vi "Format Instrument String Command.vi"(8 "error in (no error)":errorcluster, 9 "MetaData Lookup in":variant, 10 "MetaData":dbl[](array[numeric]), 11 "Command Parameters":T1) -> (0 "error out":errorcluster, 1 "MetaData Lookup out":variant, 3 "Command":string)   [LabVIEW 2019, in "Instrument Addon Engine.lvlib"]
uses:
  Instrument Addon Engine.lvlib
  Shared/Types/Command Parameters.ctl
  Shared/Types/Linked Channel Cluster.ctl
  Shared/Types/Meta Data RT Configuration Cluster.ctl
  Shared/Types/MetaData Parameters.ctl
  Shared/Types/Protocol Data Type.ctl
  Shared/Types/Metadata Channel Type.ctl
  Shared/Types/Type Cast Type.ctl
  Shared/Types/Endian.ctl
  Shared/Instrument Addon Shared.lvlib
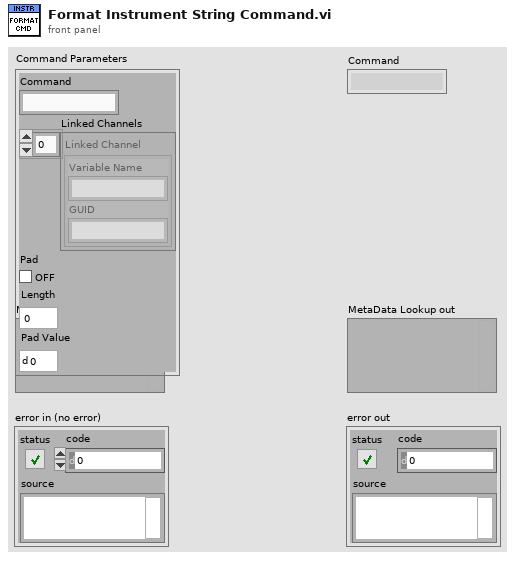
[diagram p1: front panel]
types:
  T1 = typedef "Instrument Addon Shared.lvlib/Command Parameters.ctl" = cluster{"Command":string, "Linked Channels":T2[], "Pad":bool, "Length":u32, "Pad Value":u8}
  T2 = typedef "Instrument Addon Shared.lvlib/Linked Channel Cluster.ctl" = cluster{"Variable Name":string, "GUID":string}
  T3 = typedef "Instrument Addon Shared.lvlib/Meta Data RT Configuration Cluster.ctl" = cluster{"MetaData Parameters":T4, "Data Index":i32, "Data Length":i32}
  T4 = typedef "Instrument Addon Shared.lvlib/MetaData Parameters.ctl" = cluster{"Data Type":T5, "Channel Type":T6, "List":string[], "Format String":string, "Type":T7, "Delimiter":string, "Endian":T8}
  T5 = typedef "Instrument Addon Shared.lvlib/Protocol Data Type.ctl" = enum16{"Single Channel", "Array"}
  T6 = typedef "Instrument Addon Shared.lvlib/Metadata Channel Type.ctl" = enum16{"Enumerated List", "Format", "Type Cast"}
  T7 = typedef "Instrument Addon Shared.lvlib/Type Cast Type.ctl" = enum16{"DBL", "SGL", "U64", "U32", "U16", "U8", "I64", "I32", "I16", "I8"}
  T8 = typedef "Instrument Addon Shared.lvlib/Endian.ctl" = enum16{"Native", "Little", "Big"}
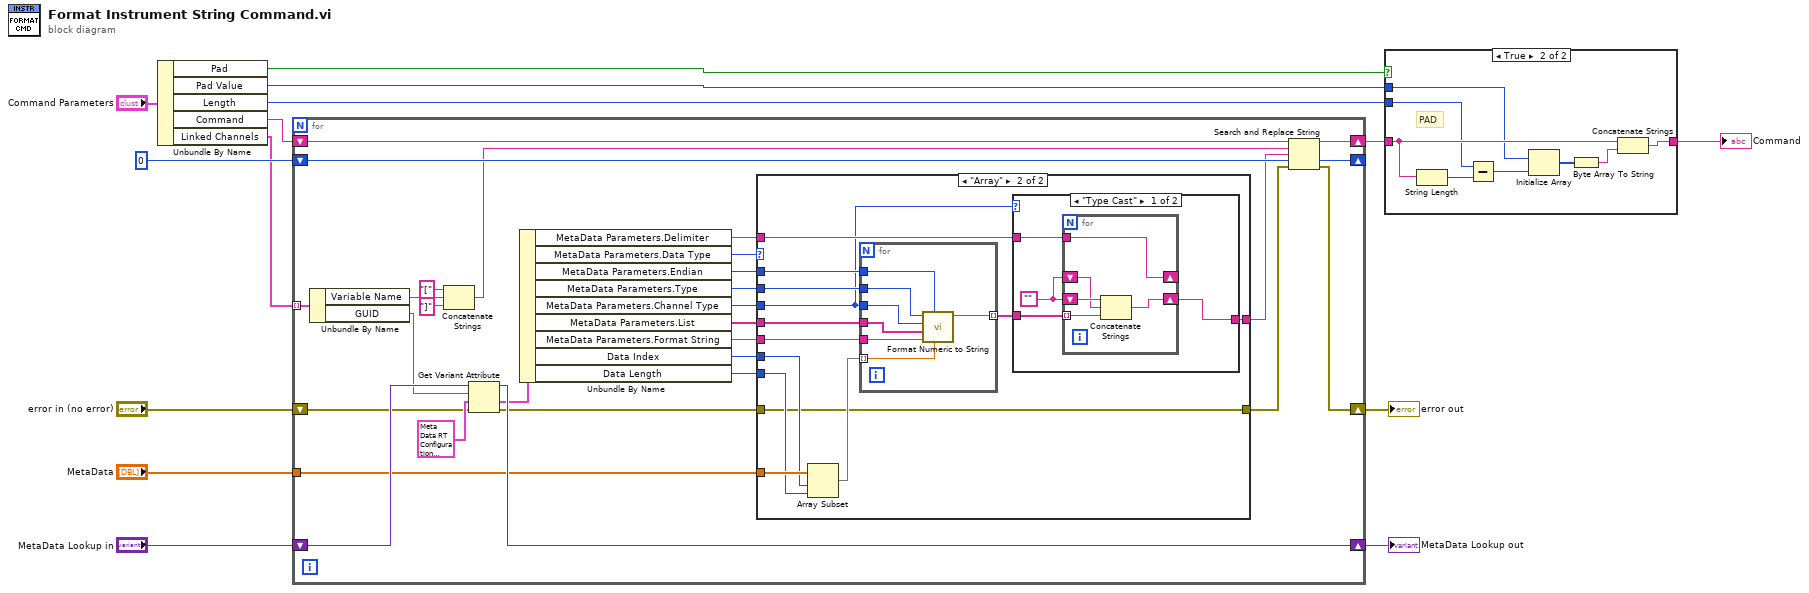
[diagram p0: block diagram]
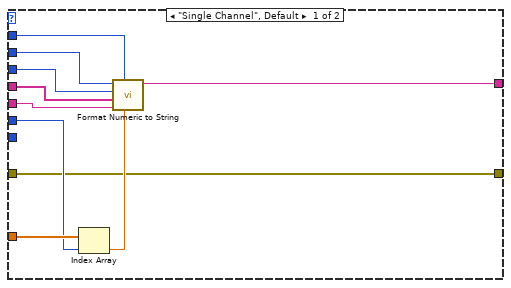
[diagram p3: hidden frame]
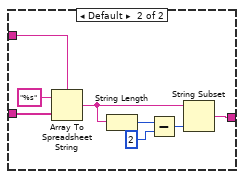
[diagram p4: hidden frame]
diagram:
  n1 = Unbundle By Name("Command Parameters") -> ("Pad"=w2:bool, "Pad Value"=w1:u8, "Length"=w3:u32, "Command"=w11:string, "Linked Channels"=w7:T2[])
  n2 = for {
    tunnel: w7 -> [w43] mode=indexing
    shift-right: [w39] -> w10
    shift-left: "MetaData Lookup in" -> [w42]
    shift-right: [w31] -> w14
    shift-left: "error in (no error)" -> [w40]
    shift-right: [w29] -> w5
    shift-left: w11 -> [w32]
    tunnel: "MetaData" -> [w22]
    shift-right: [w30] -> _
    shift-left: 0 -> [w34]
    n3 = Unbundle By Name(w43) -> ("Variable Name"=w36:string, "GUID"=w24:string)
    n4 = Concatenate Strings("[" ("string"), w36, "]" ("string")) -> (w33:string)
    n5 = Get Variant Attribute(Variant=w42, name=w24, default value (empty Variant)=T3 {"MetaData Parameters"={"Data Type"=enum."Single Channel", "Channel Type"=enum."Enumerated List", "List"=[], "Format String"="", "Type"=enum."DBL", "Delimiter"="", "Endian"=enum."Native"}, "Data Index"=0, "Data Length"=0}, error in=w40) -> (duplicate Variant=w39:variant, value=w38:T3, error out=w16:errorcluster)  [unwired: 1 out]
    n6 = Unbundle By Name(w38) -> ("MetaData Parameters.Delimiter"=w18:string, "MetaData Parameters.Data Type"=w19:T5, "MetaData Parameters.Endian"=w15:T8, "MetaData Parameters.Type"=w23:T7, "MetaData Parameters.Channel Type"=w28:T6, "MetaData Parameters.List"=w26:string[], "MetaData Parameters.Format String"=w27:string, "Data Index"=w21:i32, "Data Length"=w20:i32)
    n7 = case shown="\"Array\"" w19 {
      tunnel: w28 -> [w48 w54]
      tunnel: w27 -> [w50 w66]
      tunnel: w26 -> [w49 w65]
      tunnel: [w46 w56] -> w25
      tunnel: w23 -> [w47 w64]
      tunnel: w22 -> [w53 w63]
      tunnel: w21 -> [w52 w62]
      tunnel: w20 -> [_ w61]
      tunnel: w18 -> [_ w58]
      tunnel: [w45 w57] -> w17
      tunnel: w16 -> [w45 w57]
      tunnel: w15 -> [w44 w55]
      frame "Single Channel", Default {
        n8 = Index Array(array=w53, index=w52) -> (element=w51:dbl)
        n9 = call "Format Numeric to String.vi"("Numeric"=w51, "Endian"=w44, "Format String"=w50, "List"=w49, "Channel Type"=w48, "Type"=w47) -> ("Value"=w46:string)  [unwired: 5 in]
      }
      frame "Array" {
        n10 = Array Subset(array=w63, index=w62, length=w61) -> (w60:dbl[])
        n11 = for {
          tunnel: w54 -> [w90]
          tunnel: w66 -> [w86]
          tunnel: w65 -> [w89]
          tunnel: [w88] -> w59 mode=indexing
          tunnel: w64 -> [w87]
          tunnel: w60 -> [w85] mode=indexing
          tunnel: w55 -> [w84]
          n12 = call "Format Numeric to String.vi"("Numeric"=w85, "Endian"=w84, "Format String"=w86, "List"=w89, "Channel Type"=w90, "Type"=w87) -> ("Value"=w88:string)  [unwired: 5 in]
        }
        n13 = case shown="\"Type Cast\"" w54 {
          tunnel: w59 -> [w70 w83]
          tunnel: w58 -> [w67 w82]
          tunnel: [w69 w76] -> w56
          frame "Type Cast" {
            w68 = ""
            n14 = for {
              tunnel: w70 -> [w75] mode=indexing
              shift-right: [w74] -> w69
              shift-left: w68 -> [w73]
              shift-right: [w71] -> _
              shift-left: w68 -> [w72]
              tunnel: w67 -> [w71]
              n15 = Concatenate Strings(w73, w72, w75) -> (w74:string)
            }
          }
          frame Default {
            n16 = Array To Spreadsheet String(delimiter (Tab)=w82, array=w83, 3:"%s" ("format string")) -> (spreadsheet string=w77:string)
            n17 = String Length(string=w77) -> (length=w78:i32)
            n18 = Subtract(x=w78, y=2) -> (x-y=w80:i32)
            n19 = String Subset(string=w77, length (rest)=w80) -> (substring=w76:string)  [unwired: 1 in]
          }
        }
      }
    }
    n20 = Search and Replace String(input string=w32, search string=w33, replace string=w25, offset=w34, error in=w17) -> (result string=w29:string, offset past replacement=w30:i32, error out=w31:errorcluster)  [unwired: 3 in, 1 out]
  }
  "error out" <- w14
  "MetaData Lookup out" <- w10
  n21 = case shown="True" w2 {
    tunnel: w5 -> [w91 w96]
    tunnel: [w91 w94] -> w4
    tunnel: w3 -> [_ w93]
    tunnel: w1 -> [_ w92]
    frame False {
    }
    frame True {
      # "PAD"
      n22 = String Length(string=w96) -> (length=w99:i32)
      n23 = Subtract(x=w93, y=w99) -> (x-y=w98:u32)
      n24 = Initialize Array(w92, w98) -> (w97:u8[])
      n25 = Byte Array To String(unsigned byte array=w97) -> (string=w95:string)
      n26 = Concatenate Strings(w96, w95) -> (w94:string)
    }
  }
  "Command" <- w4
